vi "Main.vi"(11 "Module Admin":refnum<class "Delacor_lib_QMH_Module Admin.lvclass">) -> ()   [LabVIEW 2020, in "Database.lvlib"]
doc: "This template is based off of the Queued Message Handler design pattern and the Queued Message Handler project template that ships with LabVIEW.\n\nThe main difference is that the queue is private to this module and communication between modules is performed via Broadcast and Request events.\n\nRequest events are wrapped in public API methods and are handled in the Event Handling Loop (EHL) of this VI. Any module can register for Broadcast events sent by this module. The EHL generates messages based on user interface actions.\n\nThe Message Handling Loop (MHL) processes messages generated by the EHL, or by other messages. The messages are string values, so new messages can be added easily to the Message Cases case structure in the MHL. Each message cluster can also provide an optional value for Message Data, which is a variant that can be converted to whatever message-specific data is required.\n_____\nBased on Delacor QMH Project Template 5.0.0.82."
uses:
  Database.lvlib
  <vilib>/Delacor/Delacor QMH/Libraries/Module Admin_class/Delacor_lib_QMH_Module Admin.lvclass
  Module Data--cluster.ctl
  Stop Argument--cluster.ctl
  <vilib>/Delacor/Delacor QMH/Libraries/Message Queue_class/Delacor_lib_QMH_Message Queue.lvclass/Delacor_lib_QMH_Message Queue.ctl
  <vilib>/Delacor/Delacor QMH/Libraries/Module Admin_class/Delacor_lib_QMH_Module Admin.lvclass/Delacor_lib_QMH_Module Admin.ctl
  Database info Argument--cluster.ctl
  config database Argument--cluster.ctl
  Save Argument--cluster.ctl
  <vilib>/Utility/miscctls.llb/LVPointTypeDef.ctl
  <vilib>/Delacor/Delacor QMH/Libraries/Message Queue_class/Delacor_lib_QMH_Enqueue Message (Single).vi
  <vilib>/Delacor/Delacor QMH/Libraries/Module Admin_class/Delacor_lib_QMH_Get External Launch.vi
  <vilib>/addons/database/Connection.llb/DB Tools Open Connec (String).vi
  <vilib>/Utility/error.llb/Error Cluster From Error Code.vi
  <vilib>/ErrorRing/Error Ring.xnode
  <vilib>/Delacor/Delacor QMH/Libraries/Message Queue_class/Delacor_lib_QMH_Message Queue.lvclass
  <vilib>/addons/database/NI_Database_API.lvlib
  Mensajes/Mensajes.lvlib
panel:
  out "error out":errorcluster
  out "Status":string
types:
  T1 = typedef "Database.lvlib/Request Events--cluster.ctl" = cluster{"Stop Module":refnum<user-event>, "Show Panel":refnum<user-event>, "Hide Panel":refnum<user-event>, "Get Module Execution Status":refnum<user-event>, "Show Diagram":refnum<user-event>, "Database info":refnum<user-event>, "config database":refnum<user-event>, "Save":refnum<user-event>}
  T2 = typedef "Database.lvlib/Module Data--cluster.ctl" = cluster{"DB":cluster{"usuario":string, "Letra":string, "Color":string, "Codigo":string}, "Config DB":enum32{"Item 0", "Item 1"}}
  T3 = typedef "LVPointTypeDef.ctl" = cluster{"Horizontal":i16, "Vertical":i16}
  T4 = enum32{"Invalid", "Standard", "Closed", "Hidden", "Minimized", "Maximized"}
  T5 = typedef "Database.lvlib/Database info Argument--cluster.ctl" = cluster{"usuario":string, "Letra":string, "Color":string, "Forma":string}
  T6 = typedef "Database.lvlib/config database Argument--cluster.ctl" = cluster{"Config DB":enum32{"Item 0", "Item 1"}}
  T7 = typedef "Database.lvlib/Save Argument--cluster.ctl" = cluster{"Boolean":bool}
  T8 = typedef "Database.lvlib/Stop Argument--cluster.ctl" = cluster{"Origin":string, "Exit via Stop Module Req?":bool, "Wait for Module to stop?":bool}
  T9 = enum32{"invalid lock state", "Not Locked", "Locked (No Password)", "Password-protected"}
  T10 = cluster{"usuario":string, "Letra":string, "Color":string, "Codigo":string}
  T11 = typedef "NI_Database_API.lvlib/Conn ObjectReference.ctl" = refnum<k1>
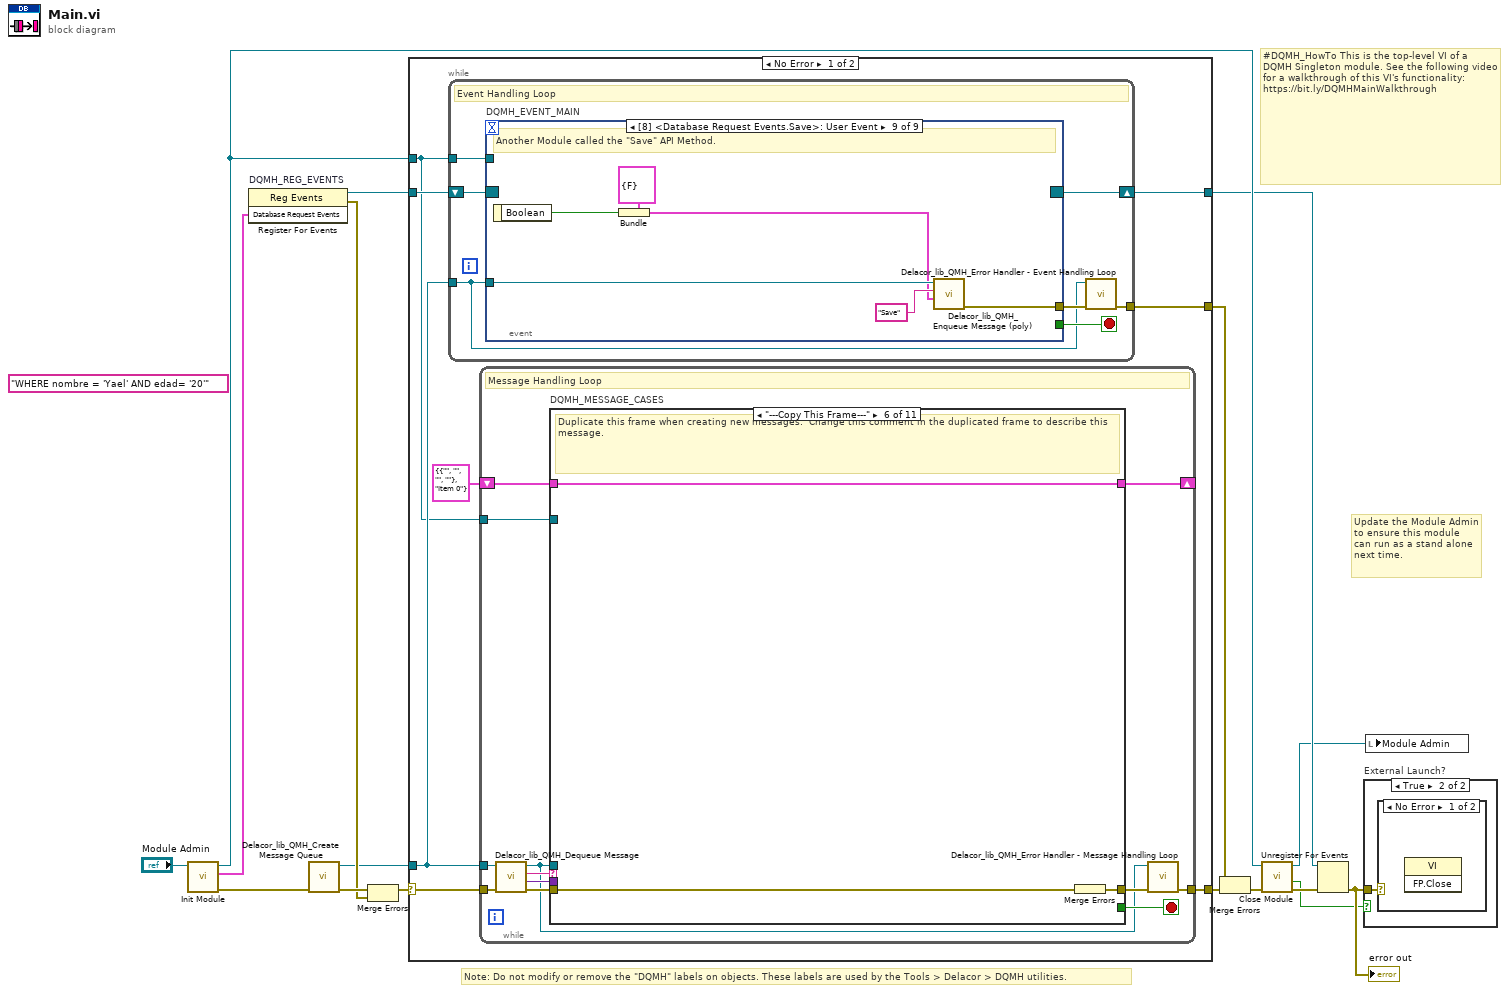
[diagram p0: block diagram]
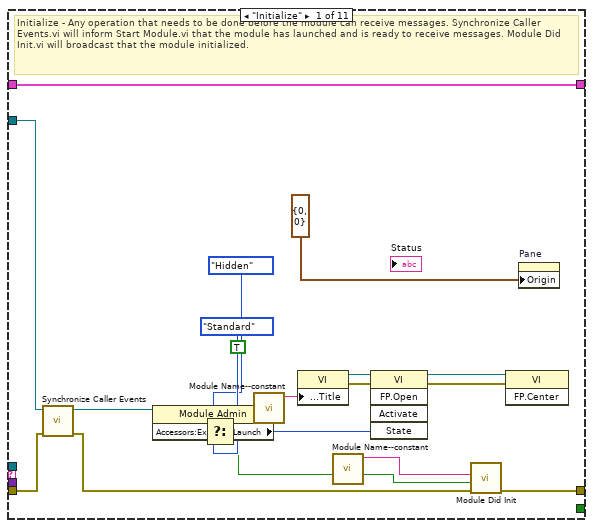
[diagram p2: hidden frame]
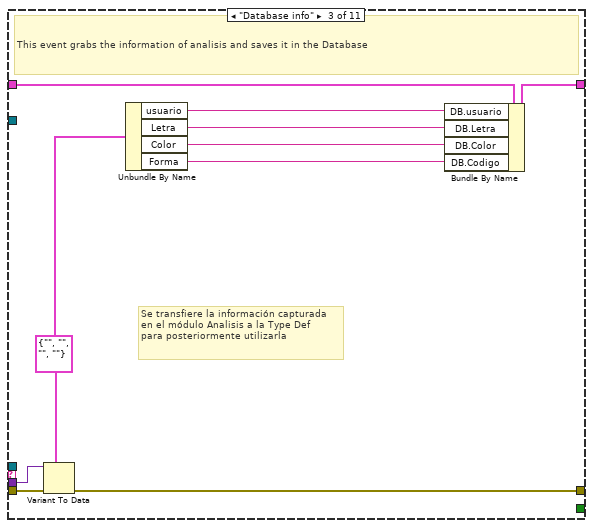
[diagram p4: hidden frame]
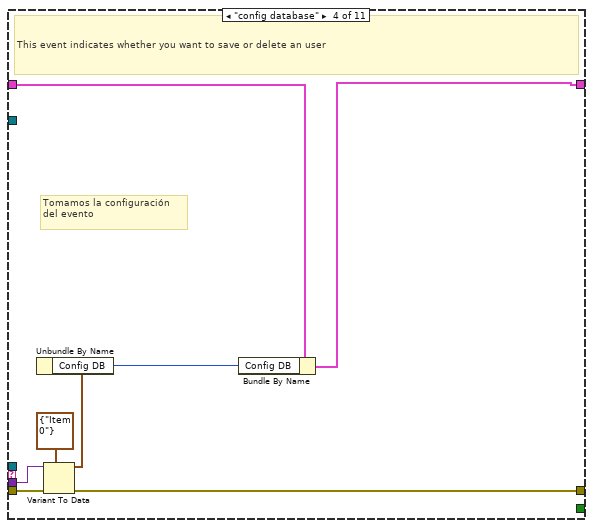
[diagram p5: hidden frame]
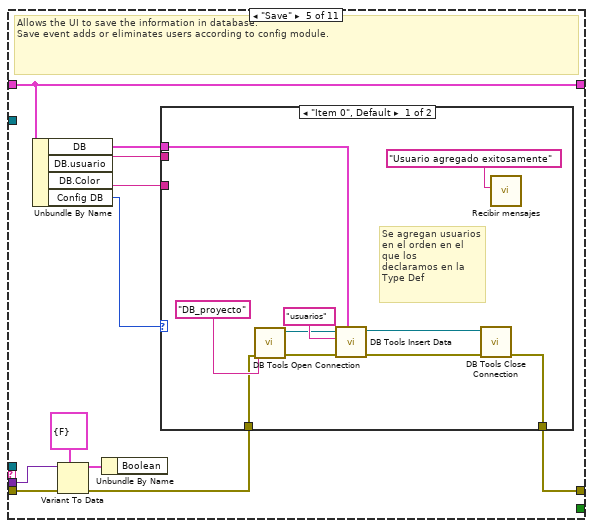
[diagram p6: hidden frame]
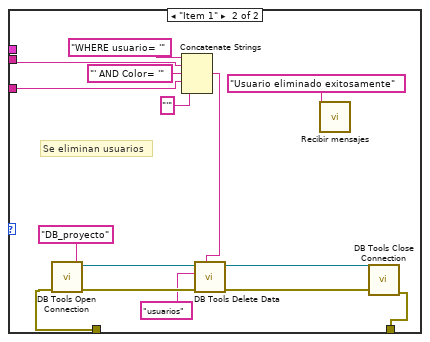
[diagram p7: hidden frame]
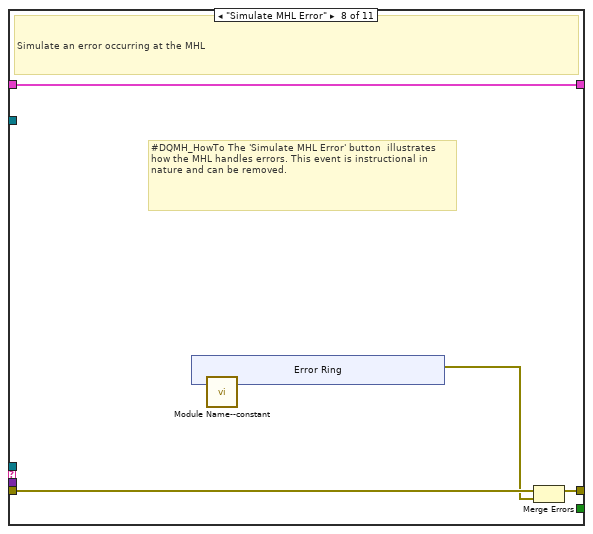
[diagram p9: hidden frame]
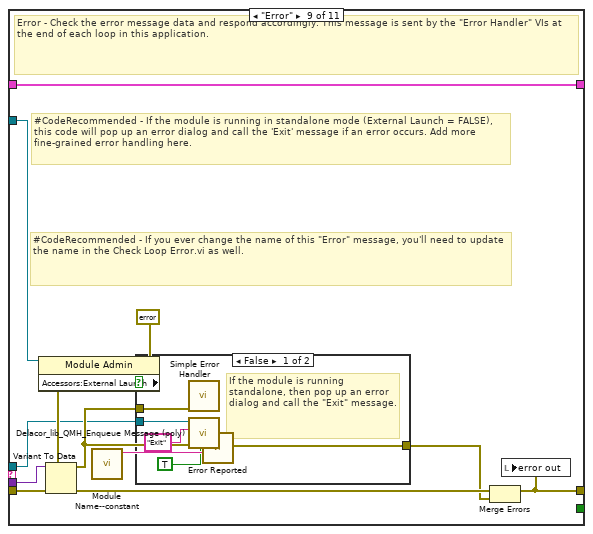
[diagram p10: hidden frame]
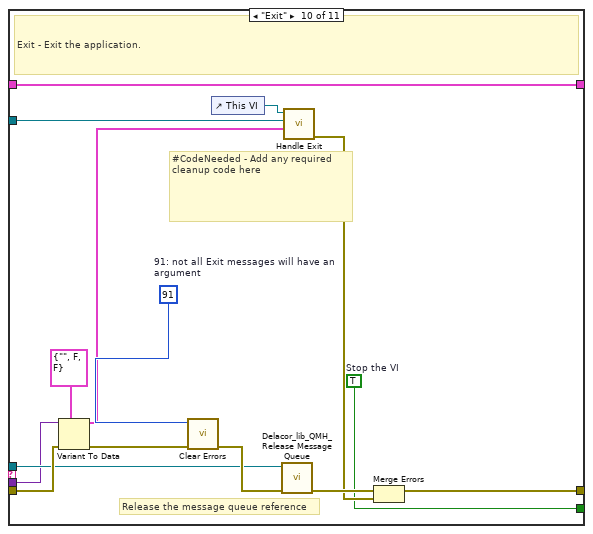
[diagram p12: hidden frame]
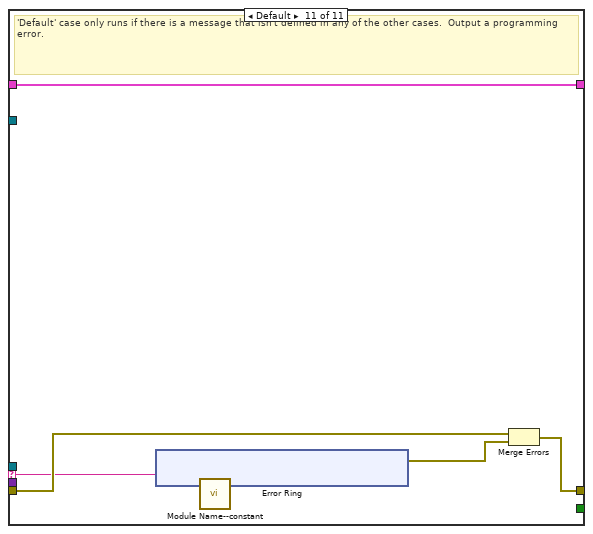
[diagram p13: hidden frame]
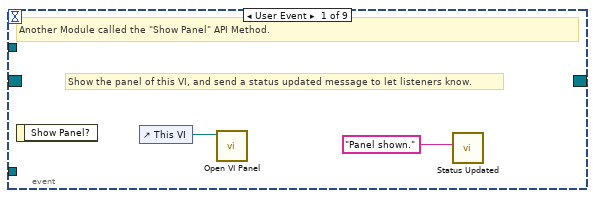
[diagram p14: hidden frame]
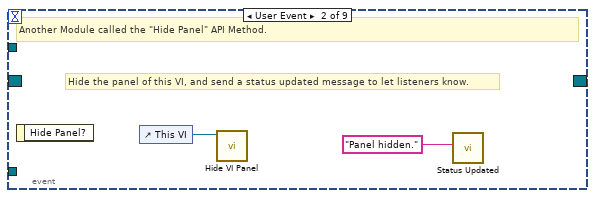
[diagram p15: hidden frame]
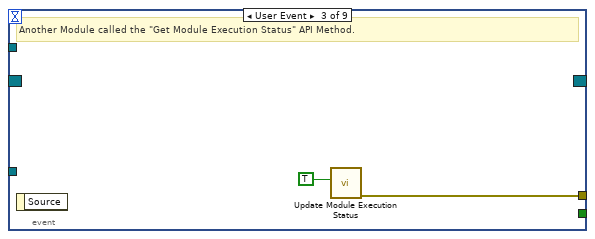
[diagram p16: hidden frame]
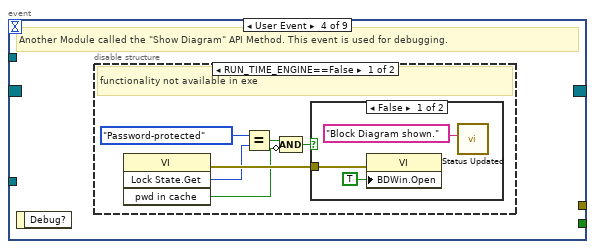
[diagram p17: hidden frame]
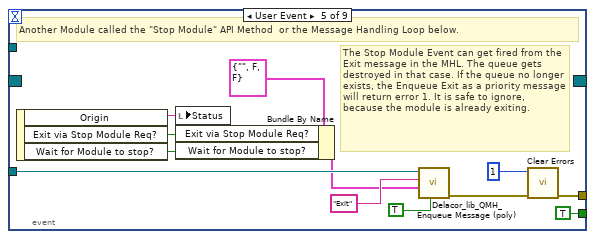
[diagram p20: hidden frame]
diagram:
  (unwired) "WHERE nombre = 'Yael' AND edad= '20'" ("condition")
  # "#DQMH_HowTo This is the top-level VI of a DQMH Singleton module. See the following video for a walkthrough of this VI's functionality: https://bit.ly/DQMHMainWalkthrough"
  # "Note: Do not modify or remove the \"DQMH\" labels on objects. These labels are used by the Tools > Delacor > DQMH utilities."
  # "Update the Module Admin to ensure this module can run as a stand alone next time."
  n1 = call "Init Module.vi"("Singleton Module Admin in"="Module Admin") -> ("error out"=w16:errorcluster, "Database Request Events"=w1:T1, "Singleton Module Admin out"=w8:refnum<class "Delacor_lib_QMH_Module Admin.lvclass">)  [unwired: 8 in]
  n2 = register-events "DQMH_REG_EVENTS"(w1) -> (reference out=w6:refnum<event-registration>, error out=w9:errorcluster)  [unwired: 2 in]
  n3 = call <vilib>:"Delacor_lib_QMH_Create Message Queue.vi"("error in (no error)"=w16) -> ("error out"=w11:errorcluster, "Message Queue"=w5:refnum<class "Delacor_lib_QMH_Message Queue.lvclass">)  [unwired: 9 in]
  n4 = Merge Errors(w11, w9) -> (w10:errorcluster)
  n5 = case shown="No Error" w10 {
    selector: w10 -> [w23 w243]
    tunnel: [w25 w242] -> w17
    tunnel: [w22 w248] -> w7
    tunnel: w6 -> [w20 w248]
    tunnel: w5 -> [w19 w241]
    tunnel: [w24 _] -> w14
    tunnel: w8 -> [w18 w244]
    frame No Error {
      n6 = while {
        tunnel: w19 -> [w176]
        shift-right: [w179] -> w22
        shift-left: w20 -> [w180]
        tunnel: [w181] -> w24
        tunnel: w18 -> [w177]
        stop <- w178 stop-if-true
        # "Event Handling Loop"
        n7 = event "DQMH_EVENT_MAIN" shown="[8] <Database Request Events.Save>: User Event" {
          selector: w180 -> [_ _ _ _ _ _ _ _ _]
          dyn-events: [_ _ _ _ _ _ _ _ _] -> w179
          timeout: _ -> [_ _ _ _ _ _ _ _ _]
          tunnel: [_ _ _ _ TRUE ("Discard?") _ _ _ _] -> w178
          tunnel: w176 -> [_ _ _ _ w205 w212 w228 w234 w240]
          tunnel: [_ _ w188 _ w208 w214 w220 w229 w235] -> w182
          tunnel: w177 -> [_ _ _ _ _ w211 _ _ _]
          event User Event {
            # "Show the panel of this VI, and send a status updated message to let listeners know."
            # "Another Module called the \"Show Panel\" API Method."
            n8 = event-data() -> ()  [unwired: 1 in, 1 out]
            n9 = control-ref of="This VI"() -> (w184:refnum<vi>)
            n10 = call "Open VI Panel.vi"("VI"=w184) -> ()  [unwired: 10 in, 1 out]
            n11 = call "Status Updated.vi"("Status"="Panel shown." ("format string")) -> ()  [unwired: 10 in, 1 out]
          }
          event User Event {
            # "Hide the panel of this VI, and send a status updated message to let listeners know."
            # "Another Module called the \"Hide Panel\" API Method."
            n12 = event-data() -> ()  [unwired: 1 in, 1 out]
            n13 = control-ref of="This VI"() -> (w186:refnum<vi>)
            n14 = call "Hide VI Panel.vi"("VI"=w186) -> ()  [unwired: 10 in, 1 out]
            n15 = call "Status Updated.vi"("Status"="Panel hidden." ("format string")) -> ()  [unwired: 10 in, 1 out]
          }
          event User Event {
            # "Another Module called the \"Get Module Execution Status\" API Method."
            n16 = event-data() -> ()  [unwired: 1 in, 1 out]
            n17 = call "Update Module Execution Status.vi"("Running?"=TRUE) -> ("error out"=w188:errorcluster)  [unwired: 10 in]
          }
          event User Event {
            # "Another Module called the \"Show Diagram\" API Method. This event is used for debugging."
            n18 = event-data() -> ()  [unwired: 1 in, 1 out]
            n19 = disable-structure shown="RUN_TIME_ENGINE==False" {
              frame condition #0 (active) {
                # "functionality not available in exe"
                n20 = invoke class="VI" method="Lock State.Get"() -> (error out=w194:errorcluster, "Get Lock State"=w193:T9, "pwd in cache"=w190:bool)  [unwired: 4 in, 1 out]
                n21 = Equal?(x=T9."Password-protected", y=w193) -> (x = y?=w191:bool)
                n22 = Compound Arithmetic op=AND(w191, invert w190) -> (w189:bool)
                n23 = case shown="False" w189 {
                  tunnel: w194 -> [w197 _]
                  frame False {
                    n24 = property class="VI"(error in=w197, "BDWin.Open"=TRUE ("Block Diagram Window:Open")) -> ()  [unwired: 1 in, 2 out]
                    n25 = call "Status Updated.vi"("Status"="Block Diagram shown." ("format string")) -> ()  [unwired: 10 in, 1 out]
                  }
                  frame True {
                    # "Password-protected VI, and the password is not in the cache. Do not show the diagram."
                  }
                }
              }
              frame condition #1 {
              }
            }
          }
          event User Event {
            # "The Stop Module Event can get fired from the Exit message in the MHL. The queue gets destroyed in that case. If the queue no longer exists, the Enqueue Exit as a priority message will return error 1. It is safe to ignore, because the module is already exiting."
            # "Another Module called the \"Stop Module\" API Method  or the Message Handling Loop below."
            n26 = event-data() -> ("Origin"=w204:string, "Exit via Stop Module Req?"=w200:bool, "Wait for Module to stop?"=w199:bool)  [unwired: 1 in]
            n27 = local write "Status"(w204) -> ()
            n28 = Bundle By Name(cluster=T8 {"Origin"="", "Exit via Stop Module Req?"=FALSE, "Wait for Module to stop?"=FALSE} ("Stop Argument"), "Exit via Stop Module Req?"=w200, "Wait for Module to stop?"=w199) -> (w198:T8)
            n29 = call-poly <vilib>:"Delacor_lib_QMH_Enqueue Message (poly).vi"("Priority Message? (F)"=TRUE, "Message Data"=w198, "Message"="Exit", "Message Queue in"=w205) -> ("error out"=w209:errorcluster)  [unwired: 6 in, 1 out]
            n30 = call <vilib>:"Clear Errors.vi"("error in (no error)"=w209, "specific error code to clear (0: all)"=1) -> ("error out"=w208:errorcluster)  [unwired: 4 in, 1 out]
          }
          event Panel Close? {
            w213 = TRUE  # Discard the event, the MHL is responsible for closing and stopping this VI.
            # "Hide the panel or send the 'Exit' message if the user clicks the 'X' on the module main VI panel."
            n31 = event-data() -> ()  [unwired: 1 in, 1 out]
            n32 = property class="Module Admin"(reference=w211) -> ("Accessors:External Launch"=w210:bool)  [unwired: 1 in, 2 out]
            n33 = case shown="True" w210 {
              tunnel: w212 -> [_ w218]
              tunnel: [_ w219] -> w214
              frame True {
                # "If externally launched, clicking the 'X' hides the panel, but doesn't close it."
                n34 = control-ref of="This VI"() -> (w215:refnum<vi>)
                n35 = call "Hide VI Panel.vi"("VI"=w215) -> ()  [unwired: 10 in, 1 out]
              }
              frame False {
                # "If run as a stand-alone VI, clicking the panel 'X' stops the VI."
                n36 = call-poly <vilib>:"Delacor_lib_QMH_Enqueue Message (poly).vi"("Priority Message? (F)"=TRUE, "Message"="Exit", "Message Queue in"=w218) -> ("error out"=w219:errorcluster)  [unwired: 7 in, 1 out]
              }
            }
            n37 = event-data("Discard?"=w213) -> ()  [unwired: 1 in, 1 out]
          }
          event User Event {
            # "Another Module called the \"Database info\" API Method."
            n38 = event-data() -> ("usuario"=w224:string, "Letra"=w223:string, "Color"=w222:string, "Forma"=w221:string)  [unwired: 1 in]
            n39 = Bundle(cluster=T5 {"usuario"="", "Letra"="", "Color"="", "Forma"=""} ("Database info Argument"), "usuario"=w224, "Letra"=w223, "Color"=w222, "Forma"=w221) -> (w225:T5)
            n40 = call-poly <vilib>:"Delacor_lib_QMH_Enqueue Message (poly).vi"("Message Data"=w225, "Message"="Database info", "Message Queue in"=w228) -> ("error out"=w220:errorcluster)  [unwired: 7 in, 1 out]
          }
          event User Event {
            # "Another Module called the \"config database\" API Method."
            n41 = event-data() -> ("Config DB"=w230:enum32{"Item 0", "Item 1"})  [unwired: 1 in]
            n42 = Bundle(cluster=T6 {"Config DB"=enum."Item 0"} ("config database Argument"), "Config DB"=w230) -> (w231:T6)
            n43 = call-poly <vilib>:"Delacor_lib_QMH_Enqueue Message (poly).vi"("Message Data"=w231, "Message"="config database", "Message Queue in"=w234) -> ("error out"=w229:errorcluster)  [unwired: 7 in, 1 out]
          }
          event User Event {
            # "Another Module called the \"Save\" API Method."
            n44 = event-data() -> ("Boolean"=w236:bool)  [unwired: 1 in]
            n45 = Bundle(cluster=T7 {"Boolean"=FALSE} ("Save Argument"), "Boolean"=w236) -> (w237:T7)
            n46 = call-poly <vilib>:"Delacor_lib_QMH_Enqueue Message (poly).vi"("Message Data"=w237, "Message"="Save", "Message Queue in"=w240) -> ("error out"=w235:errorcluster)  [unwired: 7 in, 1 out]
          }
        }
        n47 = call-dynamic "Delacor_lib_QMH_Error Handler - Event Handling Loop.vi"("error in (no error)"=w182, "Message Queue in"=w176) -> ("dup error in"=w181:errorcluster)  [unwired: 8 in, 1 out]
      }
      n48 = while {
        tunnel: w19 -> [w28]
        shift-right: [w32] -> _
        shift-left: T2 {"DB"={"usuario"="", "Letra"="", "Color"="", "Codigo"=""}, "Config DB"=enum."Item 0"} ("Data Cluster") -> [w33]
        tunnel: w23 -> [w36]
        tunnel: [w34] -> w25
        tunnel: w18 -> [w26]
        stop <- w31 stop-if-true
        # "Message Handling Loop"
        n49 = call-dynamic "Delacor_lib_QMH_Dequeue Message.vi"("error in (no error)"=w36, "Message Queue in"=w28) -> ("error out"=w35:errorcluster, "Message Data"=w29:variant, "Message"=w30:string, "Message Queue out"=w27:refnum<class "Delacor_lib_QMH_Message Queue.lvclass">)  [unwired: 6 in]
        n50 = case "DQMH_MESSAGE_CASES" shown="\"---Copy This Frame---\"" w30 {
          selector: w30 -> [_ _ _ _ _ _ _ _ _ _ w163]
          tunnel: w27 -> [_ _ _ _ _ _ _ _ w133 w155 _]
          tunnel: w35 -> [w53 w57 w68 w76 w87 w115 w117 w122 w140 w161 w165]
          tunnel: [w51 w57 w67 w72 w78 w114 w117 w121 w136 w158 w166] -> w37
          tunnel: w33 -> [w42 w56 w64 w71 w83 w113 w116 w119 w135 w154 w164]
          tunnel: [w42 w56 w62 w70 w83 w113 w116 w119 w135 w154 w164] -> w32
          tunnel: [_ _ _ _ _ _ _ _ _ w153 _] -> w31
          tunnel: w29 -> [_ _ w66 w75 w86 _ _ _ w134 w152 _]
          tunnel: w26 -> [w43 _ _ _ _ _ _ _ w132 w147 _]
          frame "Initialize" {
            # "Initialize - Any operation that needs to be done before the module can receive messages. Synchronize Caller Events.vi will inform Start Module.vi that the module has launched and is ready to receive messages. Module Did Init.vi will broadcast that the module initialized."
            n51 = call "Synchronize Caller Events.vi"("error in (no error)"=w53, "Singleton Module Admin in"=w43) -> ("error out"=w52:errorcluster, "Singleton Module Admin out"=w39:refnum<class "Delacor_lib_QMH_Module Admin.lvclass">)  [unwired: 8 in]
            n52 = property class="Module Admin"(reference=w39) -> ("Accessors:External Launch"=w47:bool)  [unwired: 1 in, 2 out]
            n53 = Select(t=T4."Hidden" ("State"), s=w47, f=T4."Standard" ("State")) -> (s? t:f=w44:T4)
            n54 = call "Module Name--constant.vi"() -> ("Module Name"=w50:string)  [unwired: 11 in]
            n55 = property class="VI"("Front Panel.Title"=w50) -> (reference out=w49:refnum<vi>, error out=w55:errorcluster)  [unwired: 2 in]
            n56 = call "Module Name--constant.vi"() -> ("Module Name"=w40:string)  [unwired: 11 in]
            n57 = invoke class="VI" method="FP.Open"(reference=w49, error in=w55, "State"=w44) -> (reference out=w48:refnum<vi>, error out=w54:errorcluster)  [unwired: 2 in, 3 out]
            n58 = call "Module Did Init.vi"("error in (no error)"=w52, "Initialized?"=TRUE, "Origin"=w40) -> ("error out"=w51:errorcluster)  [unwired: 8 in]
            n59 = invoke class="VI" method="FP.Center"(reference=w48, error in=w54) -> ()  [unwired: 1 in, 3 out]
            n60 = property on="Pane" class="Pane"("Origin"=T3 {"Horizontal"=0, "Vertical"=0}) -> ()  [unwired: 2 in, 2 out]
          }
          frame "--- Module Specific ---" {
            # "Separator -- The following cases handle messages specific to this Module."
          }
          frame "Database info" {
            # "Se transfiere la información capturada en el módulo Analisis a la Type Def \npara posteriormente utilizarla"
            # "This event grabs the information of analisis and saves it in the Database"
            n61 = Variant To Data(error in=w68, type=T5 {"usuario"="", "Letra"="", "Color"="", "Forma"=""} ("Database info Argument"), Variant=w66) -> (data=w63:T5, error out=w67:errorcluster)
            n62 = Unbundle By Name(w63) -> ("usuario"=w61:string, "Letra"=w60:string, "Color"=w59:string, "Forma"=w58:string)
            n63 = Bundle By Name(cluster=w64, "DB.usuario"=w61, "DB.Letra"=w60, "DB.Color"=w59, "DB.Codigo"=w58) -> (w62:T2)
          }
          frame "config database" {
            # "Tomamos la configuración del evento"
            # "This event indicates whether you want to save or delete an user"
            n64 = Variant To Data(error in=w76, type=T6 {"Config DB"=enum."Item 0"} ("config database Argument"), Variant=w75) -> (data=w73:T6, error out=w72:errorcluster)
            n65 = Unbundle By Name(w73) -> ("Config DB"=w69:enum32{"Item 0", "Item 1"})
            n66 = Bundle By Name(cluster=w71, "Config DB"=w69) -> (w70:T2)
          }
          frame "Save" {
            # "Allows the UI to save the information in database.\nSave event adds or eliminates users according to config module."
            n67 = Unbundle By Name(w83) -> ("DB"=w79:T10, "DB.usuario"=w82:string, "DB.Color"=w81:string, "Config DB"=w80:enum32{"Item 0", "Item 1"})
            n68 = Variant To Data(error in=w87, type=T7 {"Boolean"=FALSE} ("Save Argument"), Variant=w86) -> (data=w84:T7, error out=w77:errorcluster)
            n69 = Unbundle By Name(w84) -> ()  [unwired: 1 out]
            n70 = case shown="\"Item 0\", Default" w80 {
              tunnel: [w91 w102] -> w78
              tunnel: w82 -> [_ w100]
              tunnel: w81 -> [_ w99]
              tunnel: w79 -> [w89 _]
              tunnel: w77 -> [w88 w98]
              frame "Item 0", Default {
                # "Se agregan usuarios en el orden en el que los \ndeclaramos en la Type Def"
                n71 = call-poly <vilib>:"DB Tools Open Connection.vi"("error in (no error)"=w88, "connection information"="DB_proyecto" ("table")) -> ("error out"=w92:errorcluster, "connection reference"=w95:T11)  [unwired: 6 in]
                n72 = call <vilib>:"DB Tools Insert Data.vi"("data"=w89, "error in (no error)"=w92, "table"="usuarios", "connection reference"=w95) -> ("error out"=w93:errorcluster, "connection reference out"=w94:T11)  [unwired: 6 in]
                n73 = call <vilib>:"DB Tools Close Connection.vi"("error in (no error)"=w93, "connection reference"=w94) -> ("error out"=w91:errorcluster)  [unwired: 5 in]
                n74 = call "Recibir mensajes.vi"("Mensajes"="Usuario agregado exitosamente") -> ()  [unwired: 10 in, 1 out]
              }
              frame "Item 1" {
                # "Se eliminan usuarios"
                n75 = call-poly <vilib>:"DB Tools Open Connection.vi"("error in (no error)"=w98, "connection information"="DB_proyecto" ("table")) -> ("error out"=w110:errorcluster, "connection reference"=w111:T11)  [unwired: 6 in]
                n76 = Concatenate Strings("WHERE usuario= '" ("string"), w100, "' AND Color= '" ("string"), w99, "'" ("string")) -> (w103:string)
                n77 = call <vilib>:"DB Tools Delete Data.vi"("condition"=w103, "error in (no error)"=w110, "table"="usuarios", "connection reference"=w111) -> ("error out"=w107:errorcluster, "connection reference out"=w108:T11)  [unwired: 6 in]
                n78 = call "Recibir mensajes.vi"("Mensajes"="Usuario eliminado exitosamente") -> ()  [unwired: 10 in, 1 out]
                n79 = call <vilib>:"DB Tools Close Connection.vi"("error in (no error)"=w107, "connection reference"=w108) -> ("error out"=w102:errorcluster)  [unwired: 5 in]
              }
            }
          }
          frame "---Copy This Frame---" {
            # "Duplicate this frame when creating new messages.  Change this comment in the duplicated frame to describe this message."
            n80 = Merge Errors(w115) -> (w114:errorcluster)
          }
          frame "--- Exit and Error Handling---" {
            # "Separator - The following cases handle errors and exit messages."
          }
          frame "Simulate MHL Error" {
            # "#DQMH_HowTo The 'Simulate MHL Error' button  illustrates how the MHL handles errors. This event is instructional in nature and can be removed."
            # "Simulate an error occurring at the MHL"
            n81 = call "Module Name--constant.vi"() -> ("Module Name"=w118:string)  [unwired: 11 in]
            n82 = xnode "Error Ring"("parameter 0"=w118) -> ("error out"=w120:errorcluster)
            n83 = Merge Errors(w122, w120) -> (w121:errorcluster)
          }
          frame "Error" {
            # "#CodeRecommended - If you ever change the name of this \"Error\" message, you'll need to update the name in the Check Loop Error.vi as well."
            # "#CodeRecommended - If the module is running in standalone mode (External Launch = FALSE), this code will pop up an error dialog and call the 'Exit' message if an error occurs. Add more fine-grained error handling here."
            # "Error - Check the error message data and respond accordingly. This message is sent by the \"Error Handler\" VIs at the end of each loop in this application."
            n84 = property class="Module Admin"(reference=w132) -> ("Accessors:External Launch"=w131:bool)  [unwired: 1 in, 2 out]
            n85 = Variant To Data(error in=w140, type=errorcluster {"status"=FALSE, "code"=0, "source"=""} ("error constant"), Variant=w134) -> (data=w141:errorcluster, error out=w138:errorcluster)
            n86 = call "Module Name--constant.vi"() -> ("Module Name"=w130:string)  [unwired: 11 in]
            n87 = case shown="False" w131 {
              tunnel: [w146 _] -> w137
              tunnel: w133 -> [w144 _]
              tunnel: w141 -> [w145 _]
              frame False {
                # "If the module is running standalone, then pop up an error dialog and call the \"Exit\" message."
                n88 = call <vilib>:"Simple Error Handler.vi"("error in (no error)"=w145) -> ()  [unwired: 4 in, 5 out]
                n89 = call-poly <vilib>:"Delacor_lib_QMH_Enqueue Message (poly).vi"("Priority Message? (F)"=TRUE, "Message"="Exit", "Message Queue in"=w144) -> ("error out"=w146:errorcluster)  [unwired: 7 in, 1 out]
              }
              frame True {
                # "If the module was launched externally, calling the Error Reported broadcast VI is the only action performed by the \"Error\" message. The module's caller can then process the error appropriately."
              }
            }
            n90 = call "Error Reported.vi"("Additional Information"=w130, "Error"=w141) -> ()  [unwired: 9 in, 1 out]
            n91 = Merge Errors(w138, w137) -> (w136:errorcluster)
            n92 = local write "error out"(w136) -> ()
          }
          frame "Exit" {
            w151 = 91  # 91: not all Exit messages will have an argument
            w153 = TRUE  # Stop the VI
            # "Release the message queue reference"
            # "#CodeNeeded - Add any required cleanup code here"
            # "Exit - Exit the application."
            n93 = Variant To Data(error in=w161, type=T8 {"Origin"="", "Exit via Stop Module Req?"=FALSE, "Wait for Module to stop?"=FALSE} ("Stop Argument"), Variant=w152) -> (data=w149:T8, error out=w157:errorcluster)
            n94 = call <vilib>:"Clear Errors.vi"("error in (no error)"=w157, "specific error code to clear (0: all)"=w151) -> ("error out"=w160:errorcluster)  [unwired: 4 in, 1 out]
            n95 = control-ref of="This VI"() -> (w148:refnum<vi>)
            n96 = call-dynamic "Delacor_lib_QMH_Release Message Queue.vi"("error in (no error)"=w160, "Message Queue"=w155) -> ("error out"=w159:errorcluster)  [unwired: 9 in]
            n97 = call "Handle Exit.vi"("Stop Argument"=w149, "Admin in"=w147, "VI reference"=w148) -> ("error out"=w156:errorcluster)  [unwired: 7 in, 1 out]
            n98 = Merge Errors(w159, w156) -> (w158:errorcluster)
          }
          frame Default {
            # "'Default' case only runs if there is a message that isn't defined in any of the other cases.  Output a programming error."
            n99 = call "Module Name--constant.vi"() -> ("Module Name"=w162:string)  [unwired: 11 in]
            n100 = xnode "Error Ring"("parameter 0"=w163, "parameter 1"=w162) -> ("error out"=w167:errorcluster)
            n101 = Merge Errors(w165, w167) -> (w166:errorcluster)
          }
        }
        n102 = call-dynamic "Delacor_lib_QMH_Error Handler - Message Handling Loop.vi"("error in (no error)"=w37, "Message Queue in"=w27) -> ("dup error in"=w34:errorcluster)  [unwired: 8 in, 1 out]
      }
    }
    frame Error {
      # "Synchronize Caller Events.vi will inform Start Module.vi that the module has launched and will let the code calling Start Module.vi register for broadcasts and would permit the caller receive the broadcast that an error occurred at launch time."
      n103 = call-dynamic "Delacor_lib_QMH_Release Message Queue.vi"("error in (no error)"=w243, "Message Queue"=w241) -> ("error out"=w242:errorcluster)  [unwired: 9 in]
      n104 = call "Synchronize Caller Events.vi"("Singleton Module Admin in"=w244) -> ("error out"=w249:errorcluster)  [unwired: 9 in, 1 out]
      n105 = call "Module Name--constant.vi"() -> ("Module Name"=w247:string)  [unwired: 11 in]
      n106 = Format Into String(format string="An error occurred during initialization. %s is no longer running.", w247) -> (resulting string=w245:string)  [unwired: 2 in, 1 out]
      n107 = Merge Errors(w242, w249) -> (w250:errorcluster)
      n108 = call "Error Reported.vi"("Additional Information"=w245, "Error"=w250) -> ()  [unwired: 9 in, 1 out]
    }
  }
  n109 = Merge Errors(w14, w17) -> (w13:errorcluster)
  n110 = call "Close Module.vi"("error in (no error)"=w13, "Module Admin in"=w8) -> ("error out"=w15:errorcluster, "External Launch"=w2:bool, "Module Admin out"=w3:refnum<class "Delacor_lib_QMH_Module Admin.lvclass">)  [unwired: 7 in]
  n111 = Unregister For Events(event registration refnum=w7, error in=w15) -> (error out=w12:errorcluster)
  "error out" <- w12
  n112 = case "External Launch?" shown="True" w2 {
    tunnel: w12 -> [_ w251]
    frame False {
    }
    frame True {
      n113 = case shown="No Error" w251 {
        frame No Error {
          n114 = invoke class="VI" method="FP.Close"() -> ()  [unwired: 3 in, 3 out]
        }
        frame Error {
          n115 = invoke class="VI" method="FP.Open"("Activate"=TRUE ("Activate?")) -> ()  [unwired: 4 in, 5 out]
        }
      }
    }
  }
  n116 = local write "Module Admin"(w3) -> ()
